vi "FA_GetAgentConfig.vi"(8 "Error In":errorcluster) -> (0 "Error Out":errorcluster, 3 "AgentConfig":T1)   [LabVIEW 2013, in "FA_AgentConfig.lvlib"]
uses:
  FA_AgentConfig.lvlib
  FA_AgentConfig.ctl
  FA_LocalStore API/source/VI Source/FA_LSSpecialTypes.ctl
  FA_LocalStore API/source/VI Source/FA_LocalStore.lvlib
  FA_NativeTypes API/source/VI Source/FA_NativeTypes.lvlib
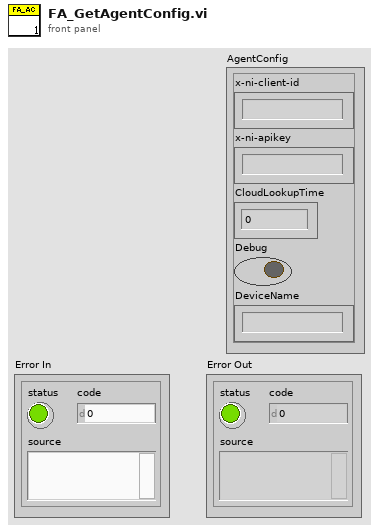
[diagram p1: front panel]
types:
  T1 = typedef "FA_AgentConfig.lvlib/FA_AgentConfig.ctl" = cluster{"x-ni-client-id":string, "x-ni-apikey":string, "CloudLookupTime":u32, "Debug":bool, "DeviceName":string}
  T2 = typedef "FA_LocalStore.lvlib/FA_LSSpecialTypes.ctl" = string
  T3 = typedef "FA_NativeTypes.lvlib/FA_Config.ctl" = cluster{"Id":string, "Name":T2, "Parameter":cluster{"Name":string, "Value":string}[], "Account":string, "CreateDate":string, "LastModified":string}
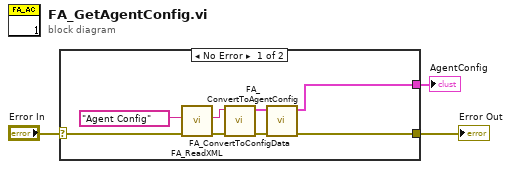
[diagram p0: block diagram]
diagram:
  n1 = case shown="No Error" "Error In" {
    selector: "Error In" -> [w10 w12]
    tunnel: [w9 w12] -> w2
    tunnel: [w4 _] -> w1
    frame No Error {
      n2 = call "FA_ReadXML.vi"("Error In"=w10, "Special Type"=T2 "Agent Config") -> ("Error Out"=w8:errorcluster, "XML String"=w5:string)  [unwired: 6 in]
      n3 = call "FA_ConvertToConfigData.vi"("Error In"=w8, "XML String"=w5) -> ("Error Out"=w7:errorcluster, "ConfigData"=w6:T3)  [unwired: 8 in]
      n4 = call "FA_ConvertToAgentConfig.vi"("Error In"=w7, "Config"=w6) -> ("Error Out"=w9:errorcluster, "AgentConfig"=w4:T1)  [unwired: 8 in]
    }
    frame Error {
    }
  }
  "Error Out" <- w2
  "AgentConfig" <- w1
